vi "子界面-查看某框和报告生成.vi"(0 "框号":dbl format="%#_13g", 1 "框组":T5(array[cluster]), 2 "反射图":T4(plugin-control), 4 "标注图":T4(plugin-control)) -> ()   [LabVIEW 2018]
uses:
  <vilib>/vision/NI_Vision_Development_Module.lvlib
panel:
  in  "返回 2":bool
  in  "报告生成":bool
  in  "反射法图像-面积阈值设置":T2(array[cluster]) {"Measurement Parameter" items=["Area"]; "下限" min=0 step=1; "上限" min=0 step=1}
  in  "穿透法图像-灰度阈值设置":T3(slide)={"Minimum Value"=0.0, "Maximum Value"=65.106384} scale=0.0..255.0
  in  "反射法图像-灰度阈值设置":T3(slide) scale=0.0..255.0
  in  "保存结果":bool
  in  "类型":string
  in  "部位":string
  in  "Color":u32[](array[colorbox])=[3381759, 16776770, 16777225, 6618880]
  in  "Overlay Type":u16[](array[ring])=[2, 1, 3, 0] items=["Rectangle", "Numbers", "Points", "Lines"]
  in  "Tab Control":T6
  out "穿透ROI":T4(plugin-control)
  out "Threshold Image":T4(plugin-control)
  out "?":T4(plugin-control)
  out "?":T4(plugin-control)
  out "Threshold Image":T4(plugin-control)
  out "Threshold Image":T4(plugin-control)
  out "Threshold Image":T4(plugin-control)
  out "穿透ROI 3":T4(plugin-control)
  out "穿透ROI 4":T4(plugin-control)
  out "反射图ROI对应区域灰度表":u32[](graph)
  out "Particle Measurements (Pixels)":dbl[][](array[numeric]) format="%.2f"
  in  "产品序号":string
  in  "测试人":string
  out "报告生成路径":path
  in  "分隔符（'\\'代码显示）":string="\t"
  in  "格式字符串":string="%f"
  out "检测结果":string[][](table)
  out "?":string
  out "面积 (pixels)":i32
  # "所选区域信息"
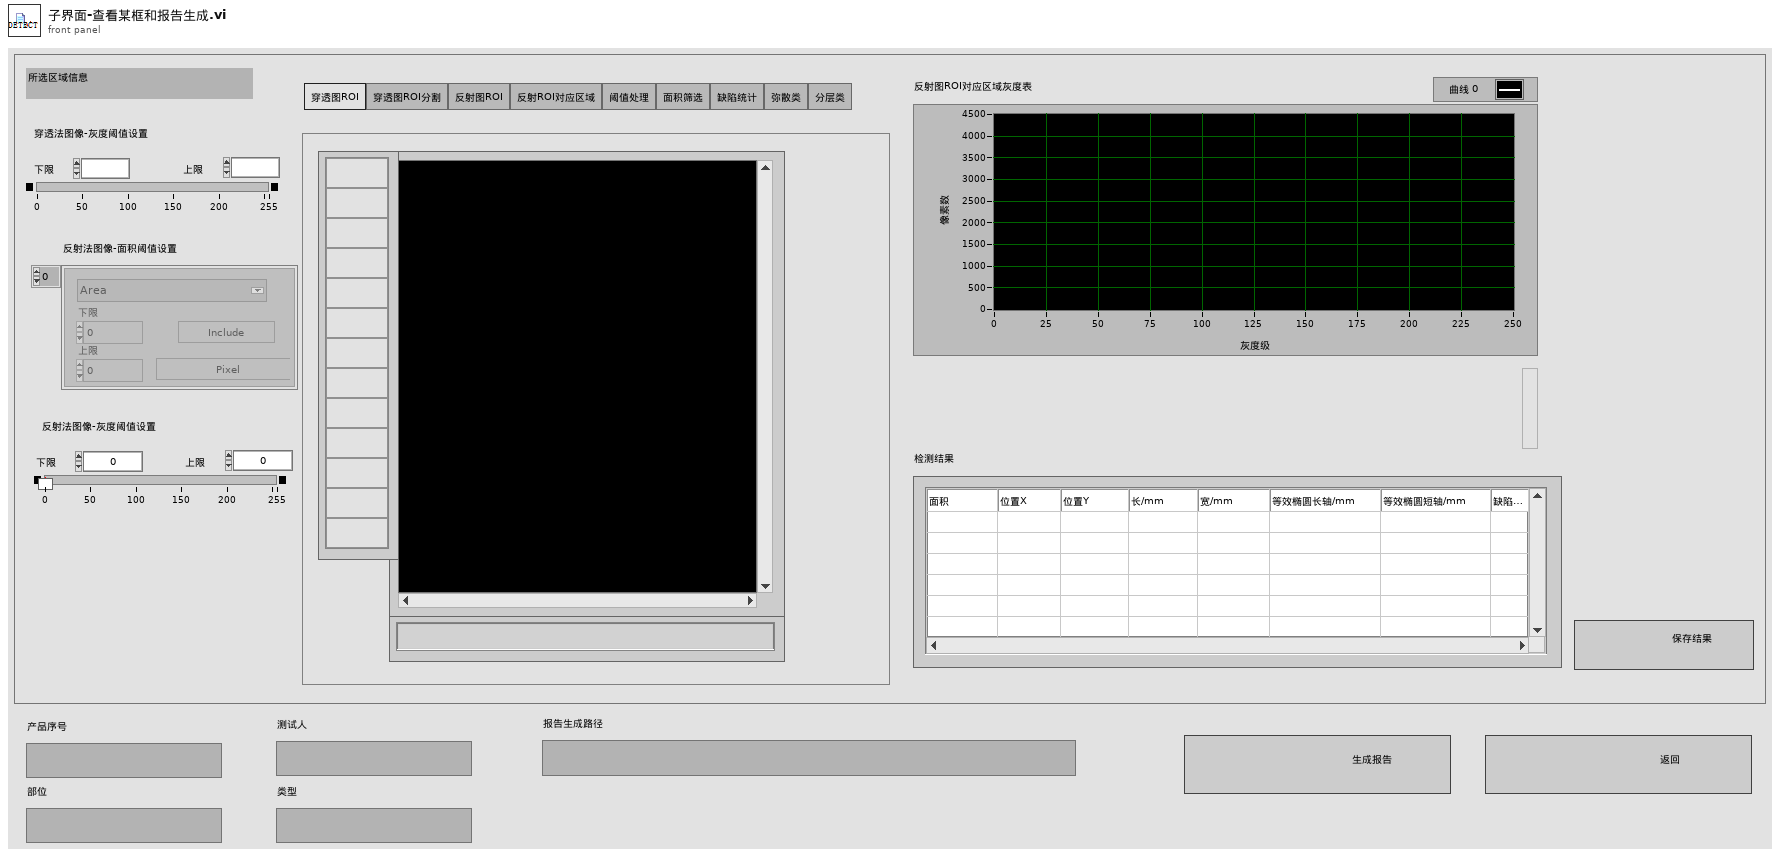
[diagram p1: front panel]
types:
  T1 = typedef "Particle Parameters" = i32
  T2 = cluster{"Measurement Parameter":T1, "下限":i32, "上限":i32, "Range":bool, "Measurement Type":bool}[]
  T3 = cluster{"Minimum Value":sgl, "Maximum Value":sgl}
  T4 = typedef "IMAQ Image.ctl" = refnum<image>
  T5 = cluster{"Global Rectangle":i32[], "Contours":cluster{"Contour Type":u32, "ROI Type":u32, "Points":i32[]}[]}[]
  T6 = typedef "控件 1.ctl" = enum32{"穿透图ROI", "穿透图ROI分割", "反射图ROI", "反射ROI对应区域", "阈值处理", "面积筛选", "缺陷统计", "弥散类", "分层类"}
  T7 = typedef "Image Type" = u32
  T8 = cluster{"Global Rectangle":i32[], "Contours":cluster{"Contour Type":u32, "ROI Type":u32, "Points":i32[]}[]}
  T9 = cluster{"反射法图像-灰度阈值设置":cluster{"Minimum Value":sgl, "Maximum Value":sgl}, "Pixel Measurements":T1[], "Overlay Type":u16[], "Color":u32[], "反射法图像-面积阈值设置":cluster{"Measurement Parameter":T1, "下限":i32, "上限":i32, "Range":bool, "Measurement Type":bool}[], "穿透法图像-灰度阈值设置":cluster{"Minimum Value":sgl, "Maximum Value":sgl}}
  T10 = cluster{"histogram":u32[], "Minimal Value":sgl, "Maximal Value":sgl, "Starting Value":sgl, "Interval Width":sgl, "Mean Value":sgl, "Standard  Variation":sgl, "Area (pixels)":i32}
  T11 = cluster{"Desired Font (Application)":enum16{"User-specified Font", "Application Font", "System Font", "Dialog Font"}, "[User-specified Font]":cluster{"Font Name":string, "Size":i16, "Strikeout?":bool, "Italic?":bool, "Underline?":bool, "Outline?":bool, "Shadow?":bool, "Bold?":bool, "Rotation Angle":dbl}, "Horizontal Alignment":i16, "Vertical Alignment":i16}
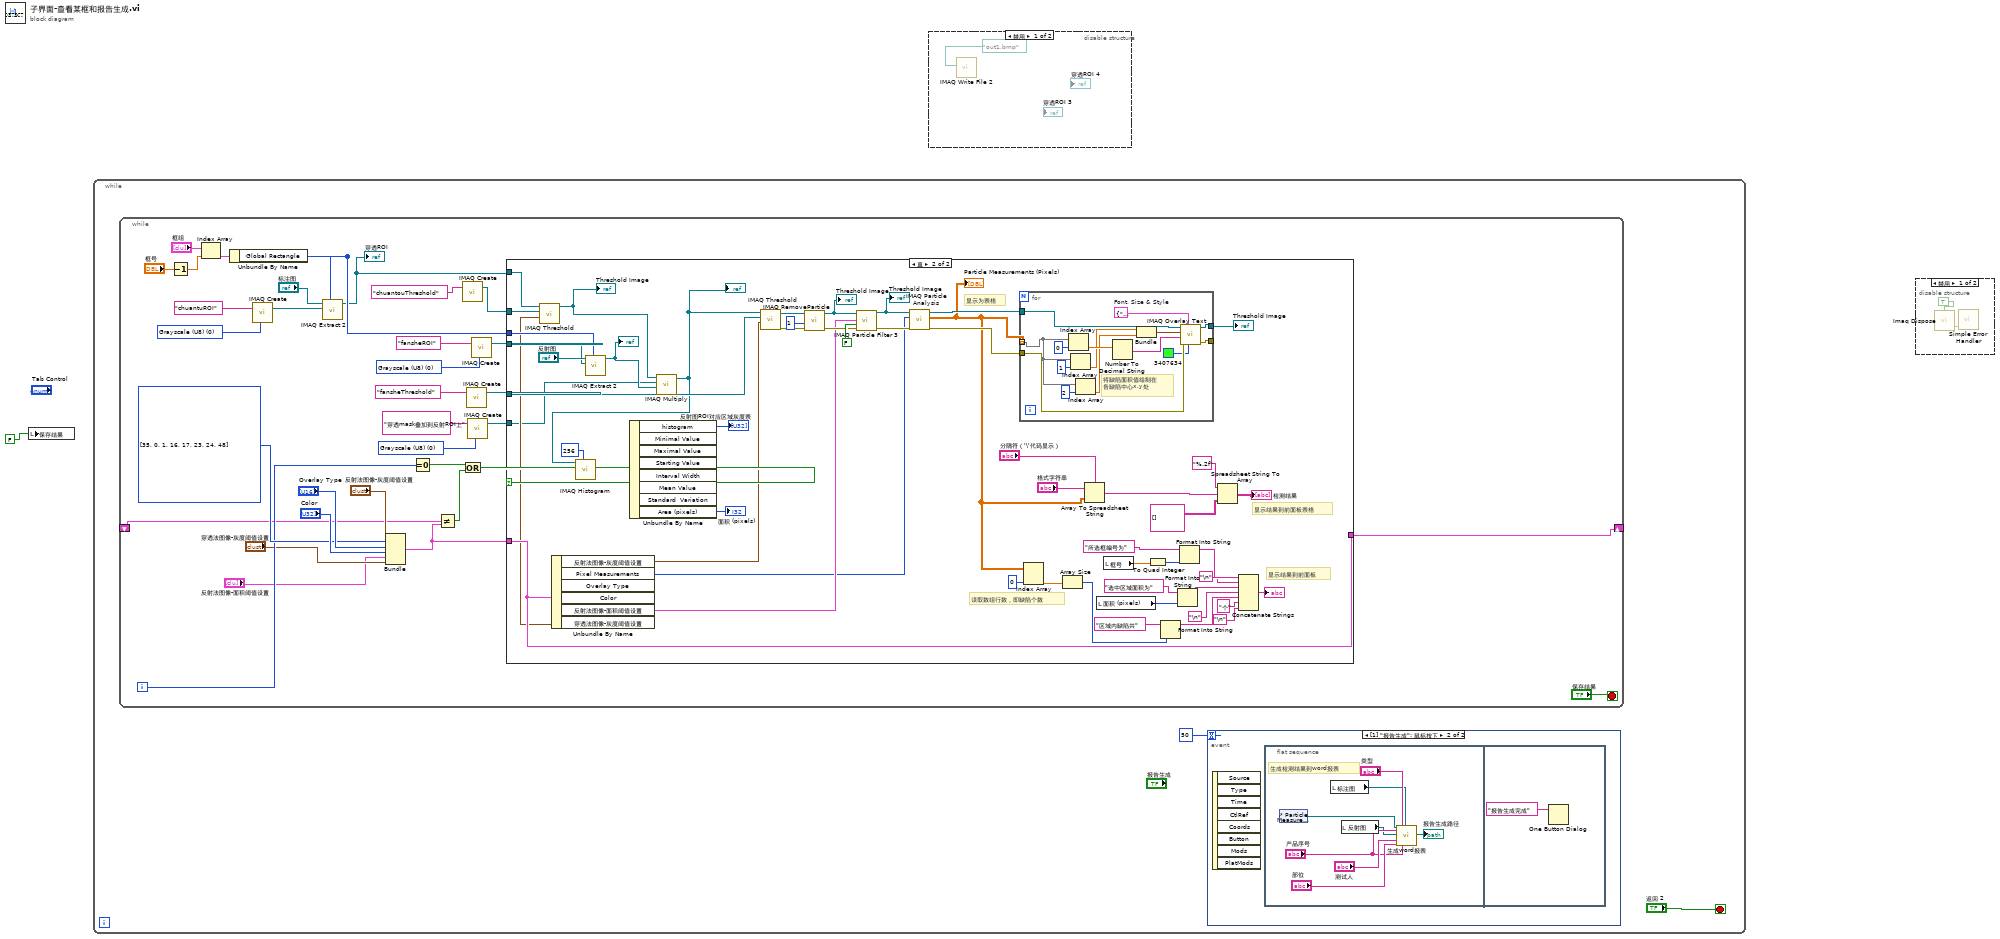
[diagram p0: block diagram]
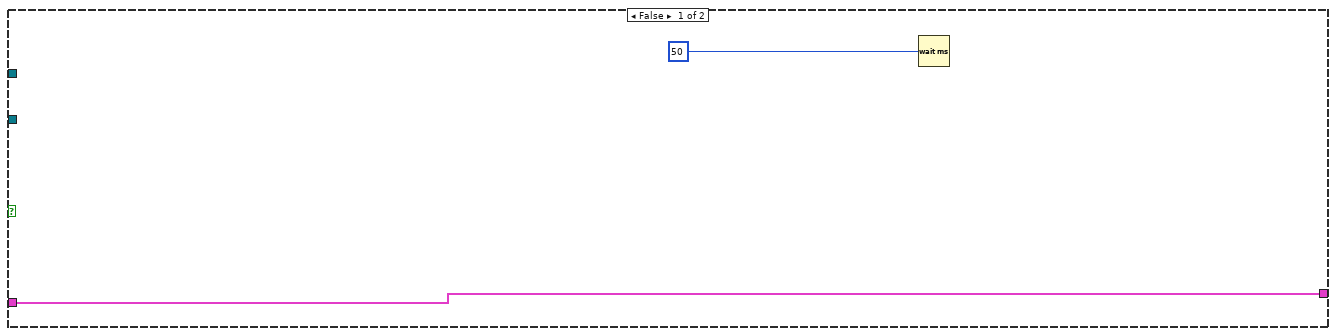
[diagram p3: hidden frame]
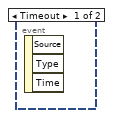
[diagram p4: hidden frame]
diagram:
  n1 = local write "保存结果"(FALSE) -> ()
  n2 = while {
    stop <- "返回 2" stop-if-true
    n3 = while {
      shift-right: [w28] -> _
      shift-left: _ -> [w27]
      i -> [w33]
      stop <- "保存结果" stop-if-true
      w5 = T7 0 items=["Grayscale (U8)", "Grayscale (I16)", "Grayscale (SGL)", "Complex (CSG)", "RGB (U32)", "HSL (U32)", "RGB (U64)", "Grayscale (U16)"] ("Image Type")
      w13 = T7 0 items=["Grayscale (U8)", "Grayscale (I16)", "Grayscale (SGL)", "Complex (CSG)", "RGB (U32)", "HSL (U32)", "RGB (U64)", "Grayscale (U16)"] ("Image Type")
      w19 = T7 0 items=["Grayscale (U8)", "Grayscale (I16)", "Grayscale (SGL)", "Complex (CSG)", "RGB (U32)", "HSL (U32)", "RGB (U64)", "Grayscale (U16)"] ("Image Type")
      w35 = T1[] [35, 0, 1, 16, 17, 23, 24, 48] items=["Center of Mass X", "Center of Mass Y", "First Pixel X", "First Pixel Y", "Bounding Rect Left", "Bounding Rect Top", "Bounding Rect Right", "Bounding Rect Bottom", "Max Feret Diameter Start X", "Max Feret Diameter Start Y", "Max Feret Diameter End X", "Max Feret Diameter End Y", "Max Horiz. Segment Length Left", "Max Horiz. Segment Length Right", "Max Horiz. Segment Length Row", "-", "Bounding Rect Width", "Bounding Rect Height", "Bounding Rect Diagonal", "Perimeter", "Convex Hull Perimeter", "Holes' Perimeter", "Max Feret Diameter", "Equivalent Ellipse Major Axis", "Equivalent Ellipse Minor Axis", "Equivalent Ellipse Minor Axis (Feret)", "Equivalent Rect Long Side", "Equivalent Rect Short Side", "Equivalent Rect Diagonal", "Equivalent Rect Short Side (Feret)", "Average Horiz. Segment Length", "Average Vert. Segment Length", "Hydraulic Radius", "Waddel Disk Diameter", "-", "Area", "Holes' Area", "Particle & Holes' Area", "Convex Hull Area", "Image Area", "-", "Number of Holes", "Number of Horiz. Segments", "Number of Vert. Segments", "-", "Orientation", "Max Feret Diameter Orientation", "-", "% Area/Image Area", "% Area/(Particle & Holes' Area)", "Ratio of Equivalent Ellipse Axes", "Ratio of Equivalent Rect Sides", "-", "Elongation Factor", "Compactness Factor", "Heywood Circularity Factor", "Type Factor", "-", "Sum X", "Sum Y", "Sum XX", "Sum XY", "Sum YY", "Sum XXX", "Sum XXY", "Sum XYY", "Sum YYY", "-", "Moment of Inertia XX", "Moment of Inertia XY", "Moment of Inertia YY", "Moment of Inertia XXX", "Moment of Inertia XXY", "Moment of Inertia XYY", "Moment of Inertia YYY", "Norm. Moment of Inertia XX", "Norm. Moment of Inertia XY", "Norm. Moment of Inertia YY", "Norm. Moment of Inertia XXX", "Norm. Moment of Inertia XXY", "Norm. Moment of Inertia XYY", "Norm. Moment of Inertia YYY", "Hu Moment 1", "Hu Moment 2", "Hu Moment 3", "Hu Moment 4", "Hu Moment 5", "Hu Moment 6", "Hu Moment 7"] ("Pixel Measurements")
      n4 = Decrement(x="框号") -> (x-1=w21:dbl)
      n5 = Index Array(array="框组", index=w21) -> (element=w23:T8)
      n6 = Unbundle By Name(w23) -> ("Global Rectangle"=w11:i32[])
      n7 = call "IMAQ Create"("Image Name"="chuantuROI", "Image Type"=w19) -> ("New Image"=w22:T4)  [unwired: 3 in, 1 out]
      n8 = call "IMAQ Extract 2"("Optional Rectangle"=w11, "Image Dst"=w22, "Image Src"="标注图") -> ("Image Dst Out"=w8:T4)  [unwired: 7 in, 1 out]
      "穿透ROI" <- w8
      n9 = Bundle("反射法图像-灰度阈值设置"="反射法图像-灰度阈值设置", "Pixel Measurements"=w35, "Overlay Type"="Overlay Type", "Color"="Color", "反射法图像-面积阈值设置"="反射法图像-面积阈值设置", "穿透法图像-灰度阈值设置"="穿透法图像-灰度阈值设置") -> (w9:T9)  [unwired: 1 in]
      n10 = Equal To 0?(x=w33) -> (x = 0?=w32:bool)
      n11 = Not Equal?(x=w27, y=w9) -> (x != y?=w31:bool)
      n12 = call "IMAQ Create"("Image Name"="chuantouThreshold") -> ("New Image"=w15:T4)  [unwired: 4 in, 1 out]
      n13 = Compound Arithmetic op=OR(w32, w31) -> (w30:bool)
      n14 = call "IMAQ Create"("Image Name"="fansheThreshold") -> ("New Image"=w10:T4)  [unwired: 4 in, 1 out]
      n15 = call "IMAQ Create"("Image Name"="穿透mask叠加到反射ROI上", "Image Type"=w5) -> ("New Image"=w4:T4)  [unwired: 3 in, 1 out]
      n16 = call "IMAQ Create"("Image Name"="fansheROI", "Image Type"=w13) -> ("New Image"=w12:T4)  [unwired: 3 in, 1 out]
      n17 = case shown="真" w30 {
        tunnel: w9 -> [w38 w52]
        tunnel: [w38 w52] -> w28
        tunnel: w15 -> [_ w61]
        tunnel: w8 -> [_ w48]
        tunnel: w12 -> [_ w59]
        tunnel: w11 -> [_ w58]
        tunnel: w10 -> [_ w57]
        tunnel: w4 -> [_ w41]
        frame False {
          n18 = Wait (ms)(milliseconds to wait=u32 50) -> ()  [unwired: 1 out]
        }
        frame True {
          # "显示结果到前面板"
          # "读取数组行数，即缺陷个数"
          # "显示结果到前面板表格"
          # "显示为表格"
          n19 = Unbundle By Name(w52) -> ("反射法图像-灰度阈值设置"=w47:T3, "Pixel Measurements"=w49:T1[], "反射法图像-面积阈值设置"=w51:T2, "穿透法图像-灰度阈值设置"=w50:T3)  [unwired: 2 out]
          n20 = call "IMAQ Threshold"("Range"=w50, "Image Dst"=w61, "Image Src"=w48) -> ("Image Dst Out"=w46:T4)  [unwired: 3 in, 5 out]
          "Threshold Image" <- w46
          n21 = call "IMAQ Extract 2"("Optional Rectangle"=w58, "Image Dst"=w59, "Image Src"="反射图") -> ("Image Dst Out"=w45:T4)  [unwired: 7 in, 1 out]
          "?" <- w45
          n22 = call "IMAQ Multiply"("Image Src A"=w46, "Image Dst"=w41, "Image Src B"=w45) -> ("Image Dst Out"=w42:T4)  [unwired: 4 in, 1 out]
          "?" <- w42
          n23 = call "IMAQ Histogram"("Number of Classes"=256, "Image"=w42) -> ("Histogram Report"=w55:T10)  [unwired: 8 in, 1 out]
          n24 = Unbundle By Name(w55) -> ("histogram"=→"反射图ROI对应区域灰度表":u32[], "Area (pixels)"=→"面积 (pixels)":i32)  [unwired: 6 out]
          n25 = call "IMAQ Threshold"("Range"=w47, "Image Dst"=w57, "Image Src"=w42) -> ("error out"=w91:errorcluster, "Image Dst Out"=w62:T4)  [unwired: 3 in, 4 out]
          n26 = call "IMAQ RemoveParticle"("error in (no error)"=w91, "Number of Erosion"=1, "Image Src"=w62) -> ("error out"=w90:errorcluster, "Image Dst Out"=w44:T4)  [unwired: 7 in]
          "Threshold Image" <- w44
          n27 = call "IMAQ Particle Filter 3"("Image Src"=w44, "Selection Values"=w51, "Keep/Remove Particles (F)"=FALSE, "error in (no error)"=w90) -> ("Image Dst Out"=w43:T4, "error out"=w89:errorcluster)  [unwired: 9 in, 1 out]
          "Threshold Image" <- w43
          n28 = call "IMAQ Particle Analysis"("error in (no error)"=w89, "Pixel Measurements"=w49, "Image"=w43) -> ("error out"=w87:errorcluster, "Particle Measurements (Pixels)"=w63:dbl[][], "Image Out (duplicate)"=w88:T4)  [unwired: 3 in, 3 out]
          "Particle Measurements (Pixels)" <- w63
          n29 = for {
            tunnel: w87 -> [w108]
            tunnel: [w107] -> _
            tunnel: [w106] -> w40
            tunnel: w88 -> [w104]
            tunnel: w63 -> [w96] mode=indexing
            w103 = T11 {"Desired Font (Application)"=enum."Application Font", "[User-specified Font]"={"Font Name"="", "Size"=12, "Strikeout?"=FALSE, "Italic?"=FALSE, "Underline?"=FALSE, "Outline?"=FALSE, "Shadow?"=FALSE, "Bold?"=FALSE, "Rotation Angle"=0.0}, "Horizontal Alignment"=0, "Vertical Alignment"=0}  # Font, Size & Style
            # "将缺陷面积值绘制在\n各缺陷中心x,y处"
            n30 = Index Array(array=w96, index=0 ("索引")) -> (element=w101:dbl)
            n31 = Index Array(array=w96, index=1 ("索引")) -> (element=w98:dbl)
            n32 = Index Array(array=w96, index=2 ("索引")) -> (element=w95:dbl)
            n33 = Number To Decimal String(number=w101) -> (decimal integer string=w102:string)  [unwired: 1 in]
            n34 = Bundle("Numeric"=w98, "Numeric"=w95) -> (w94:cluster{"Numeric":dbl, "Numeric":dbl})  [unwired: 1 in]
            n35 = call "IMAQ Overlay Text"("Text Color (black)"=u32 3407634, "Font, Size & Style"=w103, "error in (no error)"=w108, "String"=w102, "Origin"=w94, "Image"=w104) -> ("error out"=w107:errorcluster, "Image Out"=w106:T4)  [unwired: 4 in]
          }
          "Threshold Image" <- w40
          n36 = Index Array(array=w63, index (col)=0 ("禁用的索引 (列)")) -> (element=w73:dbl[])  [unwired: 1 in]
          n37 = Array Size(array=w73) -> (size(s)=w75:i32)
          n38 = Array To Spreadsheet String(delimiter (Tab)="分隔符（'\\'代码显示）", array=w63, 3:"格式字符串") -> (spreadsheet string=w83:string)
          n39 = local read "面积 (pixels)"() -> (w72:i32)
          n40 = local read "框号"() -> (w77:dbl)
          n41 = To Quad Integer(1:w77) -> (0:w76:i64)
          n42 = Format Into String(initial string="区域内缺陷共" ("初始字符串"), w75) -> (resulting string=w79:string)  [unwired: 2 in, 1 out]
          n43 = Format Into String(initial string="选中区域面积为" ("字符串"), w72) -> (resulting string=w80:string)  [unwired: 2 in, 1 out]
          n44 = Format Into String(initial string="所选框编号为" ("初始字符串"), w76) -> (resulting string=w78:string)  [unwired: 2 in, 1 out]
          n45 = Spreadsheet String To Array(format string="%.2f", spreadsheet string=w83, array type (2D Dbl)=string[][] [] ("Array")) -> (array=→"检测结果":string[][])  [unwired: 1 in]
          n46 = Concatenate Strings(w78, "\n", w80, "\n", w79, "个" ("字符串"), "\n") -> (→"?":string)
        }
      }
    }
    n47 = event shown="[1] \"报告生成\": 鼠标按下" {
      selector: _ -> [_ _]
      dyn-events: _ -> [_ _]
      timeout: 50 -> [_ _]
      event Timeout {
        n48 = event-data() -> ()  [unwired: 1 in, 3 out]
      }
      event "报告生成": Mouse Down {
        n49 = event-data() -> ()  [unwired: 1 in, 8 out]
        n50 = flat-sequence {
          frame #0 {
            # "生成检测结果到word报表"
            n51 = control-ref of="Particle Measurements (Pixels)"() -> (w114:refnum<vi>)
            n52 = local read "标注图"() -> (w109:T4)
            n53 = local read "反射图"() -> (w110:T4)
            n54 = call "生成word报表.vi"("Array输入"=w114, 1:"产品序号"="产品序号", "标注图"=w110, "测试人"="测试人", "部位"="部位", "类型"="类型", 7:"产品序号"="产品序号", "原图"=w109) -> ("报告生成路径"=→"报告生成路径":path)  [unwired: 11 in]
          }
          frame #1 {
            n55 = One Button Dialog(message="报告生成完成" ("消息")) -> ()  [unwired: 1 in, 1 out]
          }
        }
      }
    }
  }
  n56 = disable-structure shown="禁用" {
    frame Disabled {
      n57 = call-poly "IMAQ Write File 2"("File Path"=path "out1.bmp") -> ()  [unwired: 9 in, 2 out]
    }
    frame Enabled {
    }
  }
  n58 = disable-structure shown="禁用" {
    frame Disabled {
      n59 = call "Imaq Dispose"("All Images? (No)"=TRUE) -> ("error out"=w120:errorcluster)  [unwired: 5 in]
      n60 = call <vilib>:"Simple Error Handler.vi"("error in (no error)"=w120) -> ()  [unwired: 4 in, 5 out]
    }
    frame Enabled {
    }
  }
